vi "队列控制while.vi"() -> ()   [LabVIEW 2023]
panel:
  in  "Numeric":dbl
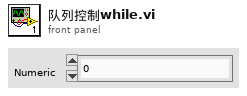
[diagram p1: front panel]
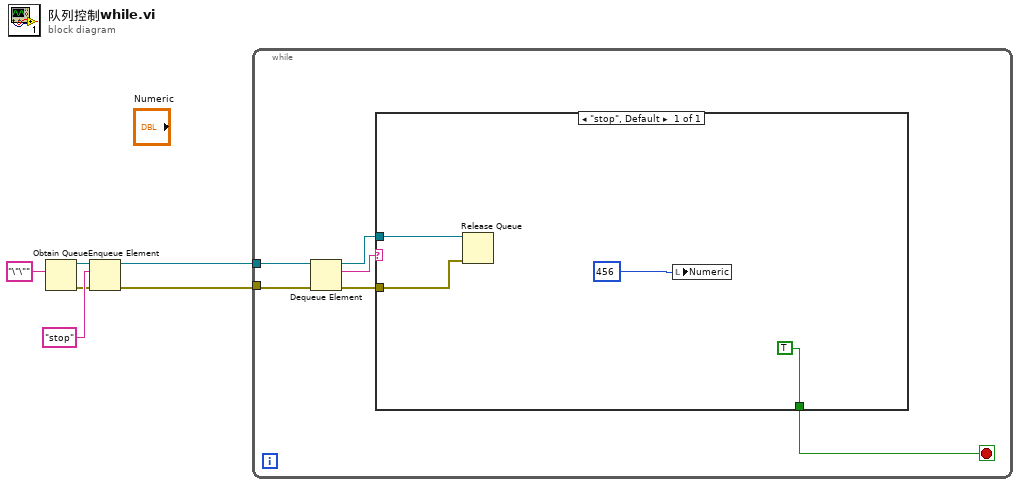
[diagram p0: block diagram]
diagram:
  n1 = Obtain Queue(element data type="\"\"") -> (queue out=w5:refnum<queue>, error out=w1:errorcluster)  [unwired: 4 in, 1 out]
  n2 = Enqueue Element(queue=w5, element="stop", error in (no error)=w1) -> (queue out=w3:refnum<queue>, error out=w2:errorcluster)  [unwired: 1 in, 1 out]
  n3 = while {
    tunnel: w3 -> [w12]
    tunnel: w2 -> [w8]
    stop <- w7 stop-if-true
    n4 = Dequeue Element(queue=w12, error in (no error)=w8) -> (queue out=w10:refnum<queue>, element=w11:string, error out=w9:errorcluster)  [unwired: 1 in, 1 out]
    n5 = case shown="\"stop\", Default" w11 {
      tunnel: w10 -> [w16]
      tunnel: w9 -> [w15]
      tunnel: [TRUE] -> w7
      frame "stop", Default {
        n6 = Release Queue(queue=w16, error in (no error)=w15) -> ()  [unwired: 1 in, 3 out]
        n7 = local write "Numeric"(456) -> ()
      }
    }
  }
